vi "TSM Relay Instrument Type ID.vi"() -> (4 "Instrument Type ID":string="Relay")   [LabVIEW 2019]
doc: "Defines the Instrument Type ID that will be referenced from the Pin Map file definition."
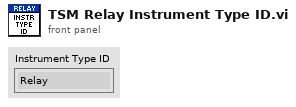
[diagram p1: front panel]
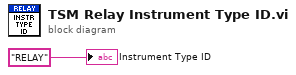
[diagram p0: block diagram]
diagram:
  "Instrument Type ID" <- "RELAY" ("Instrument Type in")
